vi "MathUtil_Interpolate.vi"(9 "T":dbl, 10 "EndValue":dbl, 11 "StartValue":dbl) -> (3 "InterpolatedValue":dbl)   [LabVIEW 2019, in "Trajectory_Library.lvlib"]
doc: "Perform linear interpolation between two values.\n \nInputs:\n - StartValue -- The value to start at.\n - EndValue -- The value to end at.\n - t -- How far between the two values to interpolate. This is clamped to [0, 1].\n\nOutputs:\n - interpolatedValue -- The interpolated value."
uses:
  Trajectory_Library.lvlib
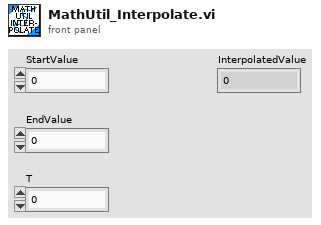
[diagram p1: front panel]
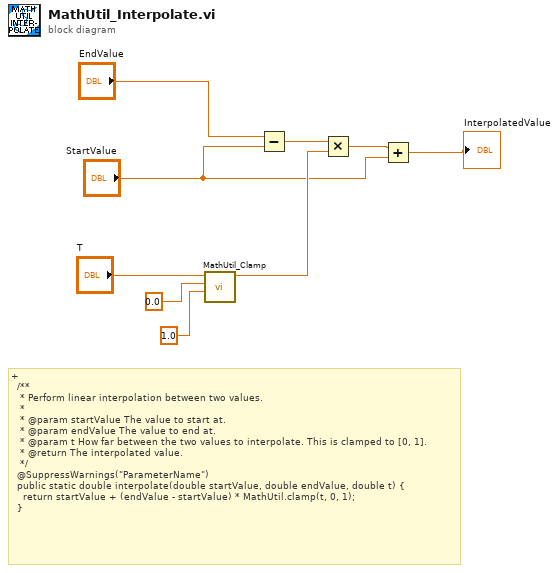
[diagram p0: block diagram]
diagram:
  # "+\n  /**\n   * Perform linear interpolation between two values.\n   *\n   * @param startValue The value to start at.\n   * @param endValue The value to end at.\n   * @param t How far between the two values to interpolate. This is clamped to [0, 1].\n   * @return The interpolated value.\n   */\n  @SuppressWarnings(\"ParameterName\")\n  public static double interpolate(double startValue, double endValue, double t) {\n    return startValue + (endValue - startValue) * MathUtil.clamp(t, 0, 1);\n  }"
  n1 = call "MathUtil_Clamp.vi"("High Limit"=1.0, "Low Limit"=0.0, "Value"="T") -> ("Result"=w4:dbl)  [unwired: 8 in]
  n2 = Subtract(x="EndValue", y="StartValue") -> (x-y=w5:dbl)
  n3 = Multiply(x=w5, y=w4) -> (x*y=w3:dbl)
  n4 = Add(x=w3, y="StartValue") -> (x+y=→"InterpolatedValue":dbl)
